vi "Points All (sub vi).vi"(9 "Boarder":i32[][](array[numeric])=[[0, 0, 18, 0], [0, 1, 18, 1], [0, 2, 18, 2], [0, 3, 18, 3], [0, 4, 18, 4], [0, 5, 18, 5], [0, 6, 18, 6], [0, 7, 18, 7], [0, 8, 18, 8], [0, 9, 18, 9], [0, 10, 18, 10], [0, 11, 18, 11], [0, 12, 18, 12], [0, 13, 18, 13], [0, 14, 18, 14], [0, 15, 18, 15], [0, 16, 18, 16], [0, 17, 18, 17], [0, 18, 18, 18], [18, 0, 19, 19], [18, 1, 0, 0], [18, 2, 0, 0], [18, 3, 0, 0], [18, 4, 0, 0], [18, 5, 0, 0], [18, 6, 0, 0], [18, 7, 0, 0], [18, 8, 0, 0], [18, 9, 0, 0], [18, 10, 0, 0], [18, 11, 0, 0], [18, 12, 0, 0], [18, 13, 0, 0], [18, 14, 0, 0], [18, 15, 0, 0], [18, 16, 0, 0], [18, 17, 0, 0], [18, 18, 0, 0], [0, 0, 0, 0], [1, 0, 0, 0], [2, 0, 0, 0], [3, 0, 0, 0], [4, 0, 0, 0], [5, 0, 0, 0], [6, 0, 0, 0], [7, 0, 0, 0], [8, 0, 0, 0], [9, 0, 0, 0], [10, 0, 0, 0], [11, 0, 0, 0], [12, 0, 0, 0], [13, 0, 0, 0], [14, 0, 0, 0], [15, 0, 0, 0], [16, 0, 0, 0], [17, 0, 0, 0], [18, 0, 0, 0], [0, 18, 0, 0], [1, 18, 0, 0], [2, 18, 0, 0], [3, 18, 0, 0], [4, 18, 0, 0], [5, 18, 0, 0], [6, 18, 0, 0], [7, 18, 0, 0], [8, 18, 0, 0], [9, 18, 0, 0], [10, 18, 0, 0], [11, 18, 0, 0], [12, 18, 0, 0], [13, 18, 0, 0], [14, 18, 0, 0], [15, 18, 0, 0], [16, 18, 0, 0], [17, 18, 0, 0], [18, 18, 0, 0], [2, 2, 0, 0], [2, 3, 0, 0], [2, 4, 0, 0], [2, 5, 0, 0], [2, 6, 0, 0], [3, 6, 0, 0], [4, 6, 0, 0], [4, 7, 0, 0], [4, 8, 0, 0], [3, 8, 0, 0], [2, 8, 0, 0], [4, 2, 0, 0], [4, 3, 0, 0], [4, 4, 0, 0], [5, 2, 0, 0], [6, 2, 0, 0], [7, 2, 0, 0], [8, 2, 0, 0], [10, 1, 0, 0], [10, 2, 0, 0], [12, 2, 0, 0], [12, 3, 0, 0], [13, 3, 0, 0], [14, 3, 0, 0], [14, 1, 0, 0], [16, 2, 0, 0], [16, 3, 0, 0], [16, 4, 0, 0], [16, 5, 0, 0], [16, 6, 0, 0], [16, 7, 0, 0], [14, 5, 0, 0], [15, 5, 0, 0], [6, 4, 0, 0], [7, 4, 0, 0], [8, 4, 0, 0], [9, 4, 0, 0], [10, 4, 0, 0], [12, 5, 0, 0], [12, 6, 0, 0], [12, 7, 0, 0], [6, 6, 0, 0], [7, 6, 0, 0], [8, 6, 0, 0], [7, 7, 0, 0], [7, 8, 0, 0], [7, 9, 0, 0], [7, 10, 0, 0], [7, 11, 0, 0], [6, 12, 0, 0], [7, 12, 0, 0], [8, 12, 0, 0], [10, 6, 0, 0], [10, 7, 0, 0], [10, 8, 0, 0], [10, 9, 0, 0], [10, 10, 0, 0], [10, 11, 0, 0], [10, 12, 0, 0], [11, 9, 0, 0], [12, 9, 0, 0], [14, 7, 0, 0], [14, 8, 0, 0], [14, 9, 0, 0], [14, 10, 0, 0], [14, 11, 0, 0], [15, 9, 0, 0], [16, 9, 0, 0], [2, 10, 0, 0], [3, 10, 0, 0], [4, 10, 0, 0], [4, 11, 0, 0], [4, 12, 0, 0], [3, 12, 0, 0], [2, 12, 0, 0], [2, 13, 0, 0], [2, 14, 0, 0], [2, 15, 0, 0], [2, 16, 0, 0], [4, 14, 0, 0], [4, 15, 0, 0], [4, 16, 0, 0], [5, 16, 0, 0], [6, 16, 0, 0], [7, 16, 0, 0], [8, 16, 0, 0], [6, 14, 0, 0], [7, 14, 0, 0], [8, 14, 0, 0], [9, 14, 0, 0], [10, 14, 0, 0], [10, 16, 0, 0], [10, 17, 0, 0], [14, 17, 0, 0], [12, 15, 0, 0], [13, 15, 0, 0], [14, 15, 0, 0], [12, 16, 0, 0], [12, 11, 0, 0], [12, 12, 0, 0], [12, 13, 0, 0], [14, 13, 0, 0], [15, 13, 0, 0], [16, 11, 0, 0], [16, 12, 0, 0], [16, 13, 0, 0], [16, 14, 0, 0], [16, 15, 0, 0], [16, 16, 0, 0]], 10 "Display":u32[][](array[colorbox])) -> (1 "Points position":i32[][](array[numeric]), 2 "Display 2":u32[][](array[colorbox]))   [LabVIEW 2014]
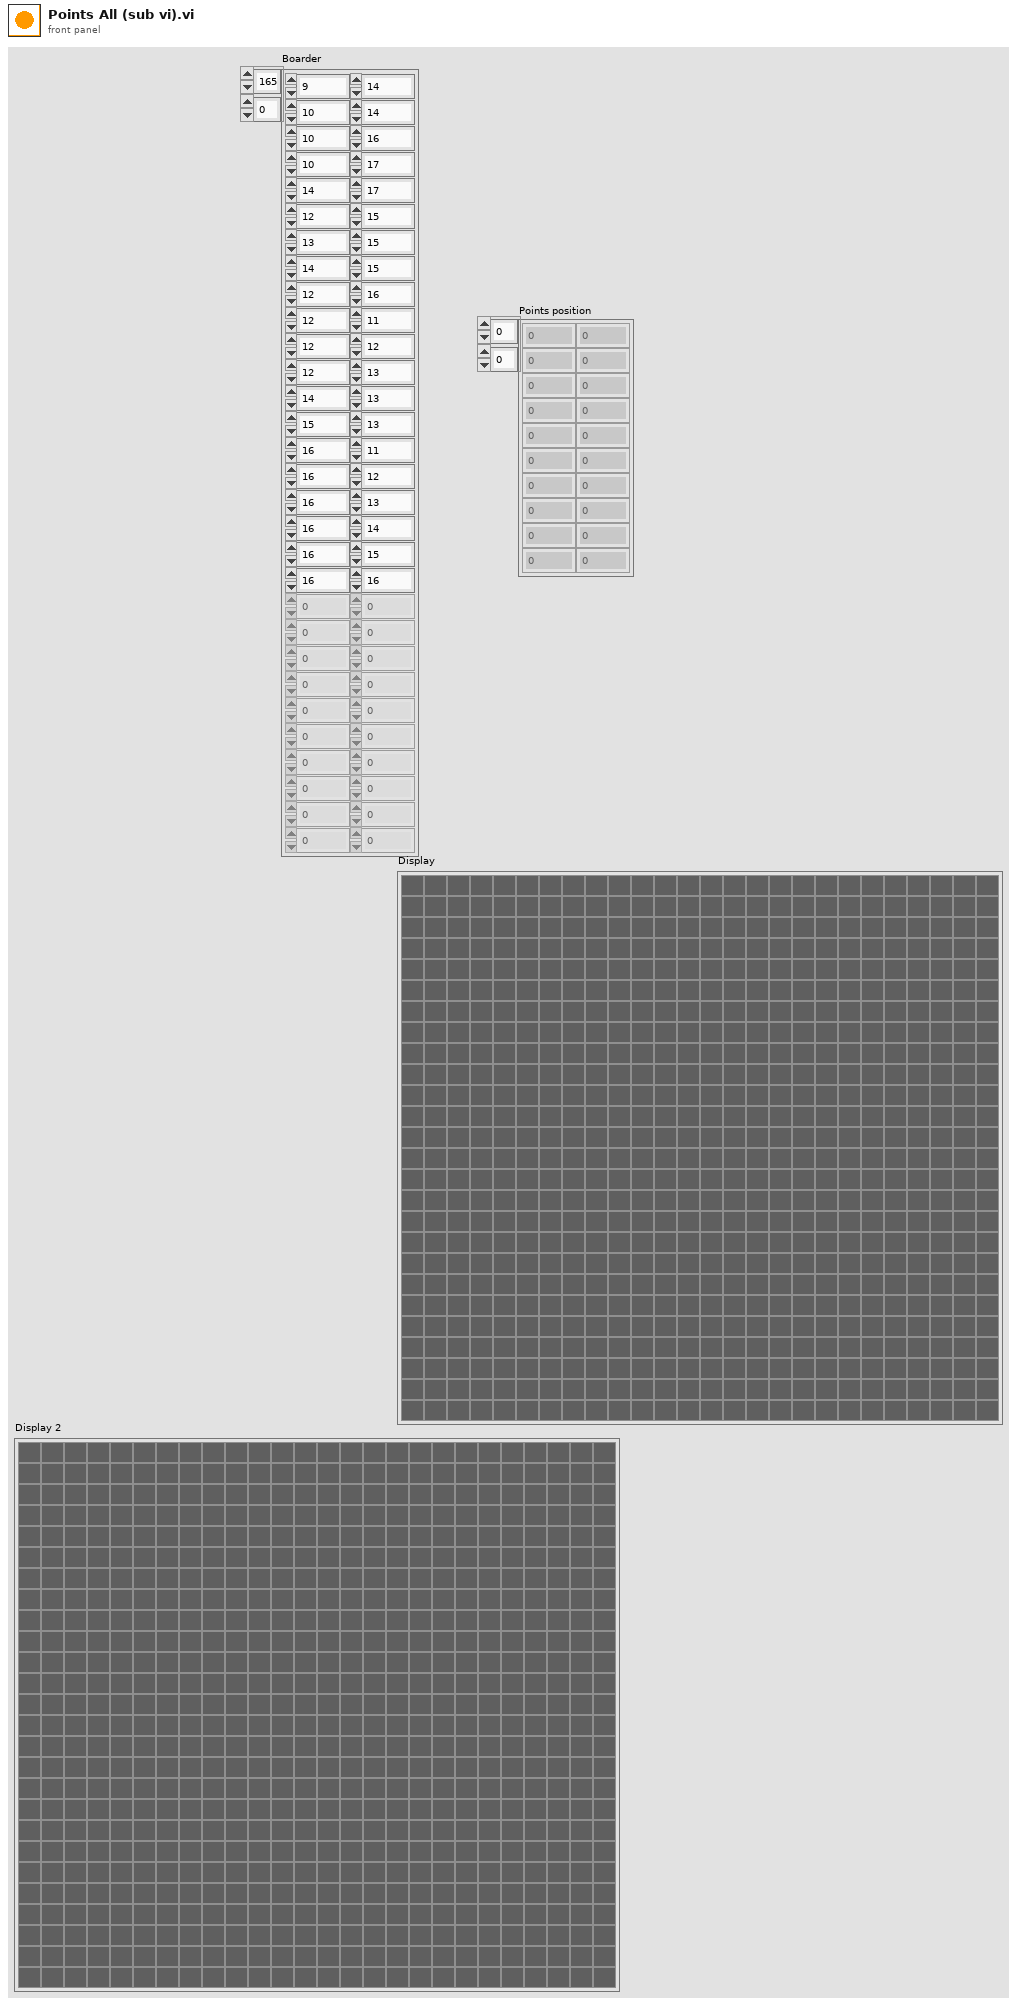
[diagram p1: front panel]
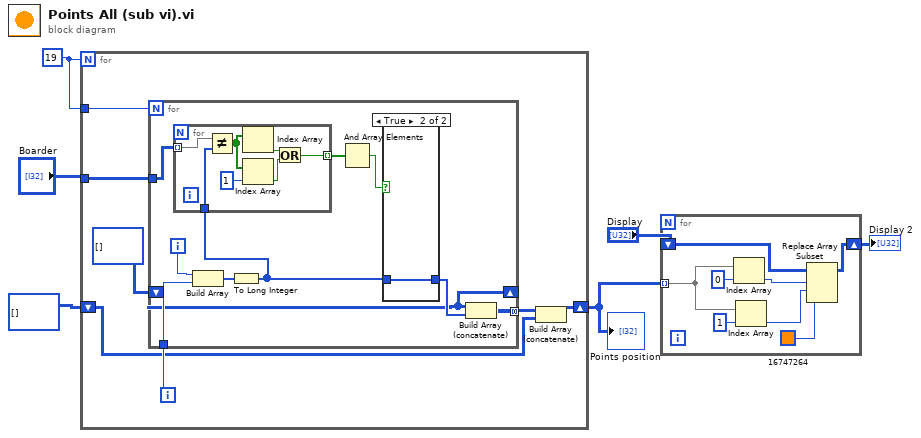
[diagram p0: block diagram]
diagram:
  w2 = 19
  n1 = for {
    N: w2 -> [_]
    shift-right: [w13] -> w4
    shift-left: i32[][] [] -> [w7]
    tunnel: w2 -> [w10]
    tunnel: "Boarder" -> [w8]
    i -> [w11]
    n2 = for {
      N: w10 -> [_]
      tunnel: w8 -> [w23]
      tunnel: [w15] -> w12 mode=concatenating
      tunnel: w11 -> [w17]
      shift-right: [w14] -> _
      shift-left: i32[][] [] -> [w14]
      i -> [w18]
      n3 = Build Array(w18, w17) -> (w22:i32[])
      n4 = To Long Integer(number=w22) -> (32bit integer=w19:i32[])
      n5 = for {
        tunnel: w23 -> [w31] mode=indexing
        tunnel: w19 -> [w26]
        tunnel: [w25] -> w21 mode=indexing
        n6 = Not Equal?(x=w31, y=w26) -> (x != y?=w30:bool[])
        n7 = Index Array(array=w30) -> (element=w27:bool)  [unwired: 1 in]
        n8 = Index Array(array=w30, index=1) -> (element=w28:bool)
        n9 = Or(x=w27, y=w28) -> (x .or. y?=w25:bool)
      }
      n10 = And Array Elements(Boolean array=w21) -> (logical AND=w20:bool)
      n11 = case shown="True" w20 {
        tunnel: w19 -> [_ w24]
        tunnel: [_ w24] -> w16
        frame False {
        }
        frame True {
        }
      }
      n12 = Build Array (concatenate)(w14, w16) -> (w15:i32[][])
    }
    n13 = Build Array (concatenate)(w12, w7) -> (w13:i32[][])
  }
  "Points position" <- w4
  n14 = for {
    shift-right: [w32] -> w3
    shift-left: "Display" -> [w33]
    tunnel: w4 -> [w34] mode=indexing
    n15 = Index Array(array=w34, index=0) -> (element=w36:i32)
    n16 = Index Array(array=w34, index=1) -> (element=w35:i32)
    n17 = Replace Array Subset(array=w33, new element=u32 16747264 ("Color Box"), index (row)=w36, index (col)=w35) -> (w32:u32[][])
  }
  "Display 2" <- w3
